vi "RRR_Inverse_Kinematics_2025.vi"() -> ()   [LabVIEW 2020]
panel:
  in  "TCP":dbl
  in  "Claw Value":dbl(slide)=1.0 scale=0.0..1.0
  in  "Scale Factor":dbl(slide)=0.7 scale=0.5..1.0
  out "RRR - Inverse Kinematics Visual":picture
  in  "Add details":bool=TRUE
  in  "Light Direction":dbl(knob)=5.611498737356196 scale format="%#.1f"
  in  "Colors":T1={"Joint 1"=16750848, "Arm 1"=16764006, "Joint 2"=26316, "Arm B"=6723993, "Joint 4"=16724787, "Claw"=16776960, "Joint 3"=26316, "Arm C"=6723993}
  in  "Elbow Up?":bool
  out "Theta_3":dbl=90.00005693440856
  out "Theta_2":dbl=59.999943065571856
  out "Theta_1":dbl=120.00000000001958
  out "Y_Target":dbl=23.3013
  out "Y_Wrist":dbl=43.3013
  out "Y_Elbow":dbl=43.30127018921338
  out "X_Target":dbl=-55.0
  out "X_Wrist":dbl=-54.99999999999999
  out "X_Elbow":dbl=-25.0000000000148
  in  "L3":dbl=20.0
  in  "Psi (Target Orientation)":dbl=270.0
  out "RRR - Inverse Kinematics":cluster{dbl[], dbl[]}(graph)={[0.0, -25.0000000000148, -54.99999999999999, -55.0], [0.0, 43.30127018921338, 43.3013, 23.3013]}
  in  "Y (Target Position)":dbl=23.3013
  in  "X (Target Position)":dbl=-55.0
  in  "L2":dbl=30.0
  in  "L1":dbl=50.0
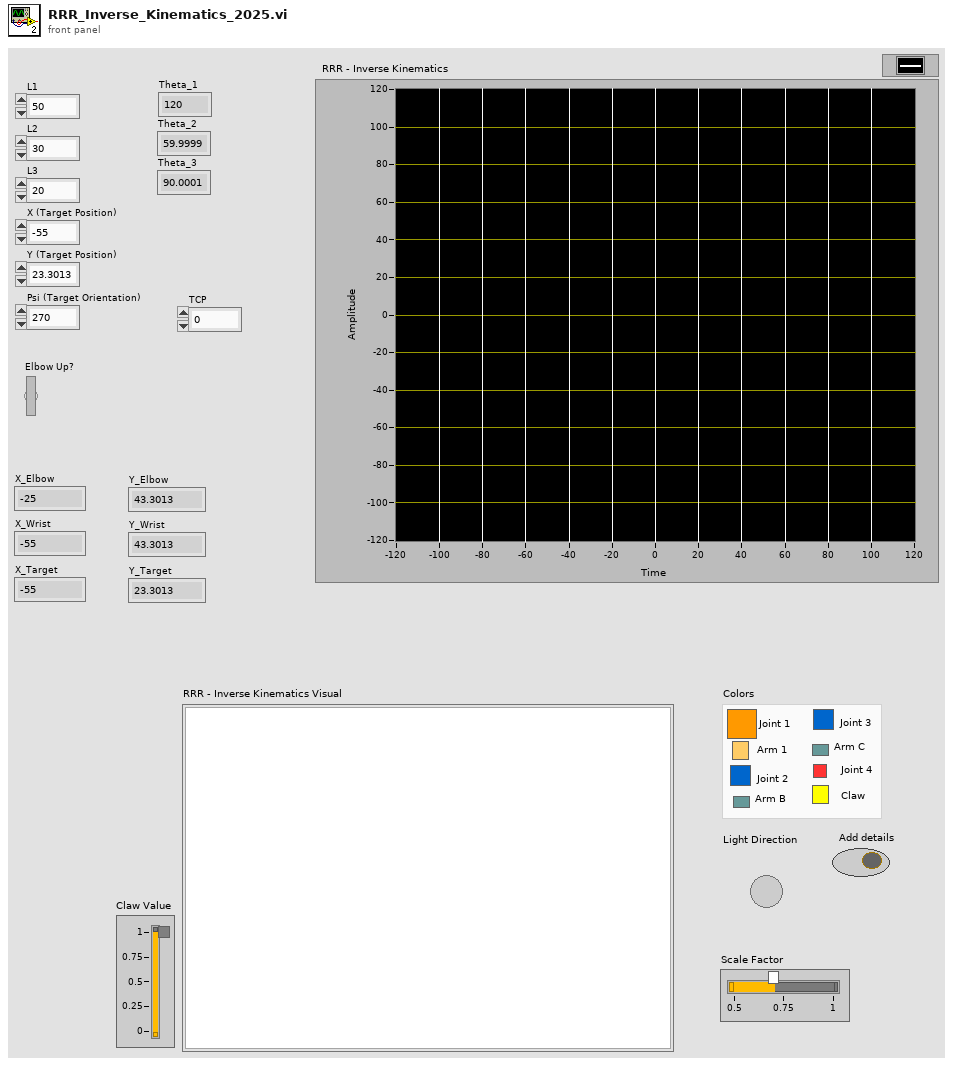
[diagram p1: front panel]
types:
  T1 = cluster{"Joint 1":u32, "Arm 1":u32, "Joint 2":u32, "Arm B":u32, "Joint 4":u32, "Claw":u32, "Joint 3":u32, "Arm C":u32}
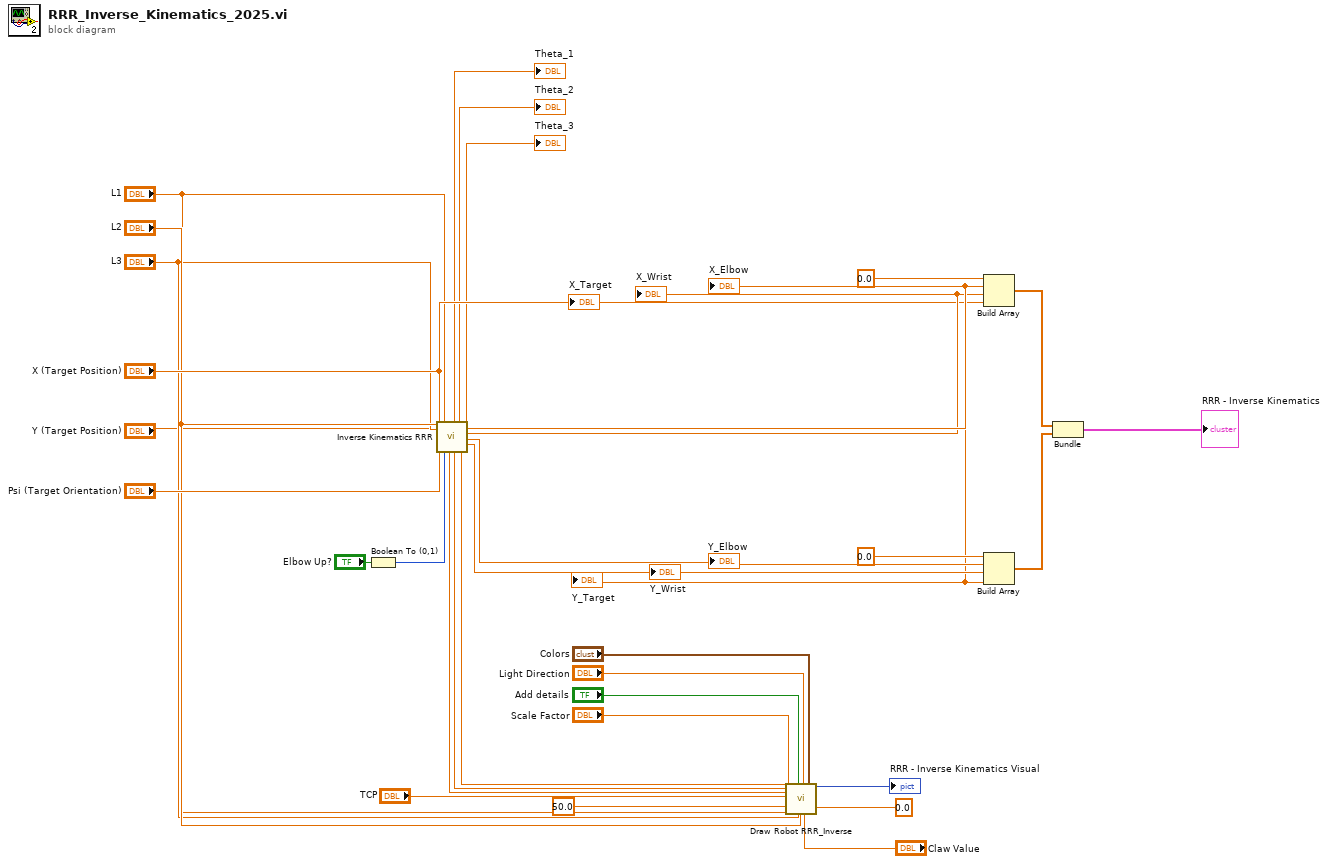
[diagram p0: block diagram]
diagram:
  n1 = Boolean To (0,1)(Boolean="Elbow Up?") -> (0, 1=w20:i16)
  n2 = call "Inverse Kinematics RRR.vi"("L2"="L2", "L3"="L3", "X (Target Position)"="X (Target Position)", "Y (Target Position)"="Y (Target Position)", "Psi (Target Orientation)"="Psi (Target Orientation)", "L1"="L1", "Numeric 4"=w20) -> ("Numeric"=w3:dbl, "th1_deg"=→"Theta_1":dbl, "Numeric 3"=w7:dbl, "th2_deg"=→"Theta_2":dbl, "Numeric 2"=w5:dbl, "th3_deg"=→"Theta_3":dbl, "x_elbow"=w31:dbl, "x_wrist"=w25:dbl, "y_elbow"=w23:dbl, "y_wrist"=w24:dbl)  [unwired: 3 in]
  "X_Elbow" <- w31
  "X_Wrist" <- w25
  "Y_Elbow" <- w23
  "Y_Wrist" <- w24
  n3 = call "Draw Robot RRR_Inverse.vi"("Scale Factor"="Scale Factor", "Numeric 3"=w7, "TCP"="TCP", "Numeric"=w3, "y 2"=50.0 ("y"), "L1"="L1", "Numeric 2"=w5, "L2"="L2", "Add details"="Add details", "L3"="L3", "Light Direction"="Light Direction", "Claw Value"="Claw Value", "Colors"="Colors", "y"=0.0) -> ("Picture Out"=→"RRR - Inverse Kinematics Visual":picture)  [unwired: 5 in]
  n4 = Build Array(0.0 ("element"), w31, w25, "X (Target Position)") -> (w29:dbl[])
  n5 = Build Array(0.0 ("element"), w23, w24, "Y (Target Position)") -> (w28:dbl[])
  n6 = Bundle(w29, w28) -> (→"RRR - Inverse Kinematics":cluster{dbl[], dbl[]})  [unwired: 1 in]
  "X_Target" <- "X (Target Position)"
  "Y_Target" <- "Y (Target Position)"
